vi "Lua Thread class path.vi"() -> (3 "Lua Thread Class Path":path)   [LabVIEW 2020, in "Lua DevUtil.lvlib"]
uses:
  Lua DevUtil.lvlib
  Lua for LabVIEW/Lua Thread/Resume.vi
  Lua for LabVIEW/Lua Thread/Lua Thread.lvclass
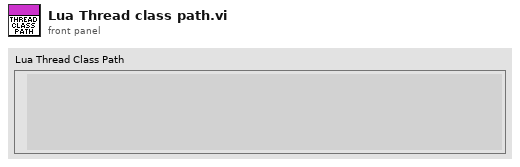
[diagram p1: front panel]
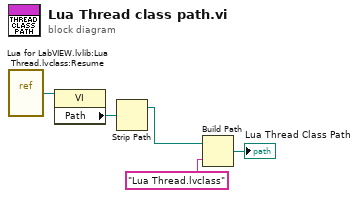
[diagram p0: block diagram]
diagram:
  n1 = vi-ref "Lua for LabVIEW.lvlib:Lua Thread.lvclass:Resume.vi"() -> (w5:refnum<vi>)
  n2 = property class="VI"(reference=w5) -> ("Path"=w4:path)  [unwired: 1 in, 2 out]
  n3 = Strip Path(path=w4) -> (stripped path=w1:path)  [unwired: 1 out]
  n4 = Build Path(base path=w1, name or relative path="Lua Thread.lvclass") -> (appended path=→"Lua Thread Class Path":path)
